vi "ANN_4WheeledController.vi"(5 "ESN trained":T1={"output to internal feedback?"=FALSE, "output to output feedback?"=FALSE, "input to output feedforward?"=TRUE, "number of input (K)"=2, "number of internal (N)"=222, "number of output (L)"=2, "input normalization vector"=[0.6006126900000001, 2.94100566], "output restore vector"=[30.199380389999998, 30.418265820000002], "input weight (N*K)"=array222x2[444 elements], "feedback weight (N*L)"=[], "internal weight (N*N)"=array222x222[49284 elements], "output weight (L*(K+N+L))"=array2x224[448 elements]}, 6 "dt":dbl, 7 "model type":T3 items=["Analytical Kinematic Model", "ANN Kinematic Model"], 8 "wref (nan)":dbl=nan, 9 "vref (nan)":dbl=nan, 10 "desired posture":T4, 11 "current posture":T4) -> (2 "wr":dbl, 3 "wl":dbl)   [LabVIEW 2017]
doc: "This VI contains the velocity controller and inverse kinematic model. The VI returns the linear velocities of the left and right wheels."
uses:
  VehiclePosture.ctl
  ModelType.ctl
  ESN network/ESN_Network.ctl
  <vilib>/Analysis/Matrix/Datatypes/RealMatrix.ctl
  <vilib>/Analysis/Matrix/NI_Matrix.lvlib
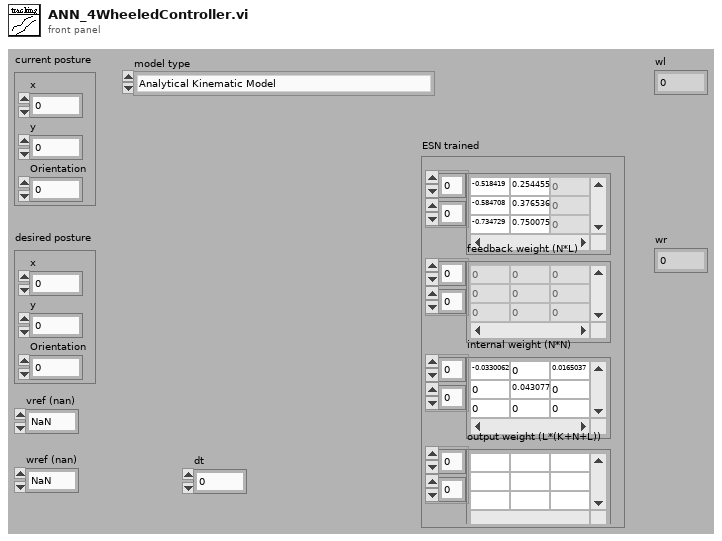
[diagram p1: front panel]
types:
  T1 = typedef "ESN_Network.ctl" = cluster{"output to internal feedback?":bool, "output to output feedback?":bool, "input to output feedforward?":bool, "number of input (K)":i32, "number of internal (N)":i32, "number of output (L)":i32, "input normalization vector":dbl[], "output restore vector":dbl[], "input weight (N*K)":T2, "feedback weight (N*L)":T2, "internal weight (N*N)":T2, "output weight (L*(K+N+L))":T2}
  T2 = typedef "NI_Matrix.lvlib/RealMatrix.ctl" = dbl[][]
  T3 = typedef "ModelType.ctl" = u16
  T4 = typedef "VehiclePosture.ctl" = cluster{"x":dbl, "y":dbl, "Orientation":dbl}
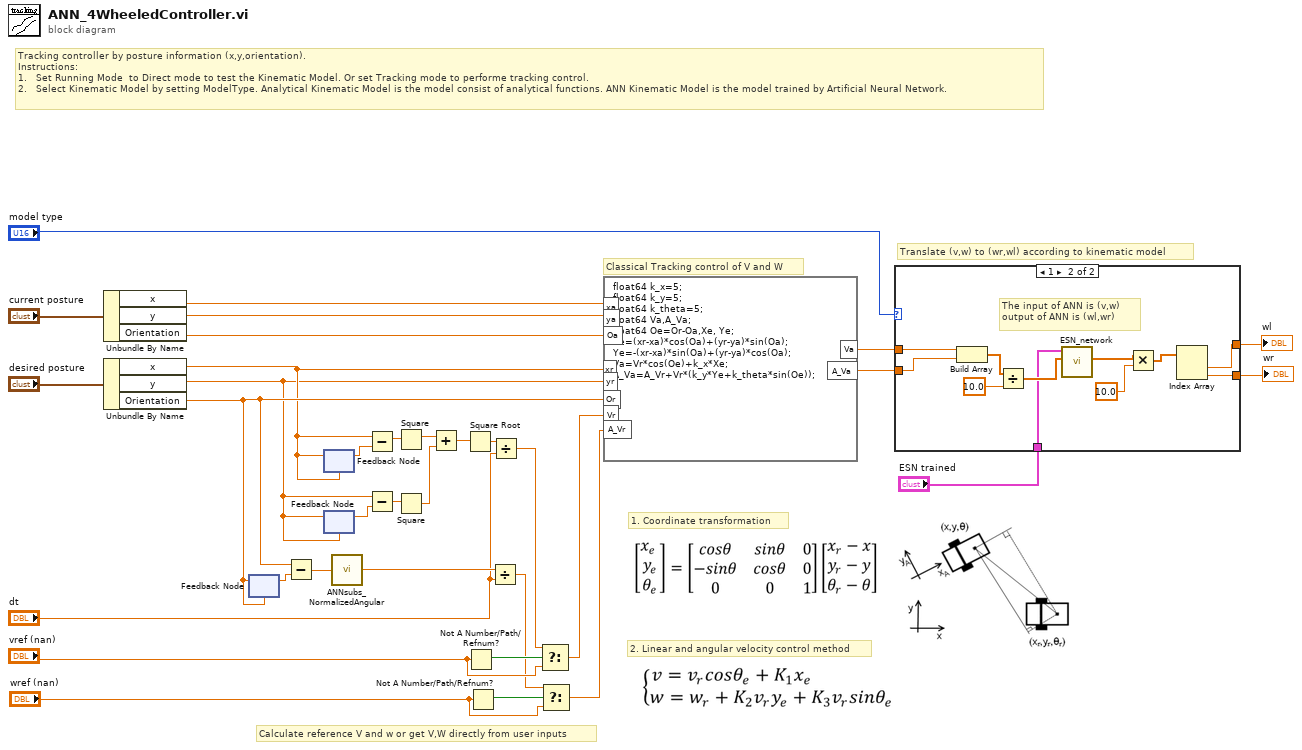
[diagram p0: block diagram]
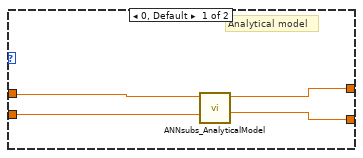
[diagram p2: hidden frame]
diagram:
  # "Translate (v,w) to (wr,wl) according to kinematic model"
  # "2.\tLinear and angular velocity control method"
  # "1.\tCoordinate transformation"
  # "Tracking controller by posture information (x,y,orientation). \nInstructions:\n1.   Set Running Mode  to Direct mode to test the Kinematic Model. Or set Tracking mode to performe tracking control.\n2.   Select Kinematic Model by setting ModelType. Analytical Kinematic Model is the model consist of analytical functions. ANN Kinematic Model is the model trained by Artificial Neural Network."
  # "Classical Tracking control of V and W"
  # "Calculate reference V and w or get V,W directly from user inputs"
  n1 = Unbundle By Name("current posture") -> ("x"=w34:dbl, "y"=w33:dbl, "Orientation"=w32:dbl)
  n2 = Unbundle By Name("desired posture") -> ("x"=w26:dbl, "y"=w24:dbl, "Orientation"=w30:dbl)
  n3 = feedback #1(w30) -> (w31:dbl)
  n4 = feedback-in #1(w30) -> ()
  n5 = Subtract(x=w30, y=w31) -> (x-y=w29:dbl)
  n6 = feedback #2(w26) -> (w27:dbl)
  n7 = feedback-in #2(w26) -> ()
  n8 = feedback #3(w24) -> (w25:dbl)
  n9 = feedback-in #3(w24) -> ()
  n10 = call "ANNsubs_NormalizedAngular.vi"("Delta angle"=w29) -> ("Delta angle out"=w28:dbl)
  n11 = Subtract(x=w26, y=w27) -> (x-y=w23:dbl)
  n12 = Subtract(x=w24, y=w25) -> (x-y=w22:dbl)
  n13 = Square(x=w23) -> (x^2=w21:dbl)
  n14 = Square(x=w22) -> (x^2=w20:dbl)
  n15 = Add(x=w21, y=w20) -> (x+y=w19:dbl)
  n16 = Square Root(x=w19) -> (sqrt(x)=w18:dbl)
  n17 = Not A Number/Path/Refnum?(number/path/refnum="vref (nan)") -> (NaN/Path/Refnum?=w14:bool)
  n18 = Not A Number/Path/Refnum?(number/path/refnum="wref (nan)") -> (NaN/Path/Refnum?=w11:bool)
  n19 = Divide(x=w28, y="dt") -> (x/y=w9:dbl)
  n20 = Divide(x=w18, y="dt") -> (x/y=w13:dbl)
  n21 = Select(t=w13, s=w14, f="vref (nan)") -> (s? t:f=w2:dbl)
  n22 = Select(t=w9, s=w11, f="wref (nan)") -> (s? t:f=w7:dbl)
  n23 = formula code="float64 k_x=5;\nfloat64 k_y=5;\nfloat64 k_theta=5;\nfloat64 Va,A_Va;\nfloat64 Oe=Or-Oa,Xe, Ye;\nXe=(xr-xa)*cos(Oa)+(yr-ya)*sin(Oa);\nYe=-(xr-xa)*sin(Oa)+(yr-ya)*cos(Oa);\nVa=Vr*cos(Oe)+k_x*Xe;\nA_Va=A_Vr+Vr*(k_y*Ye+k_theta*sin(Oe));"("xa"=w34, "ya"=w33, "Oa"=w32, "xr"=w26, "yr"=w24, "Or"=w30, "Vr"=w2, "A_Vr"=w7) -> ("Va"=w6:dbl, "A_Va"=w5:dbl)
  n24 = case shown="1" "model type" {
    tunnel: w6 -> [w36 w46]
    tunnel: w5 -> [w35 w45]
    tunnel: [w38 w40] -> w4
    tunnel: [w37 w41] -> w3
    tunnel: "ESN trained" -> [_ w39]
    frame 0, Default {
      # "Analytical model"
      n25 = call "ANNsubs_AnalyticalModel.vi"("AngularV"=w35, "linearV"=w36) -> ("W R"=w37:dbl, "W L"=w38:dbl)  [unwired: 8 in]
    }
    frame 1 {
      # "The input of ANN is (v,w)\noutput of ANN is (wl,wr)"
      n26 = Build Array(w46, w45) -> (w44:dbl[])
      n27 = Divide(x=w44, y=10.0 ("element")) -> (x/y=w42:dbl[])
      n28 = call "ESN_network.vi"("input"=w42, "ESN Status"=w39) -> ("output"=w49:dbl[])  [unwired: 6 in, 3 out]
      n29 = Multiply(x=w49, y=10.0 ("element")) -> (x*y=w47:dbl[])
      n30 = Index Array(array=w47) -> (element #1=w40:dbl, element #2=w41:dbl)  [unwired: 2 in]
    }
  }
  "wl" <- w4
  "wr" <- w3
